vi "CRC16MODBUS.vi"(8 "error in (no error)":errorcluster caption="错误输入（无错误）", 11 "In_Data":u8[](array[numeric]) format="%.0x") -> (0 "error out":errorcluster caption="错误输出", 3 "CRC16":u16 format="%.0x")   [LabVIEW 2015]
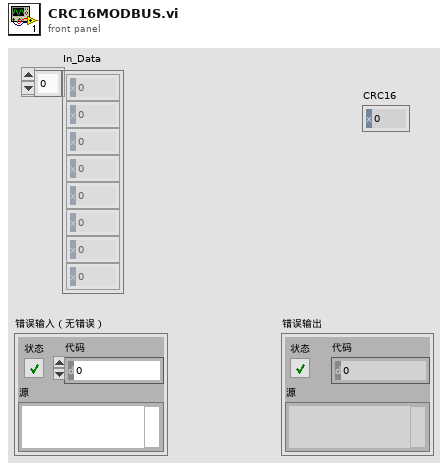
[diagram p1: front panel]
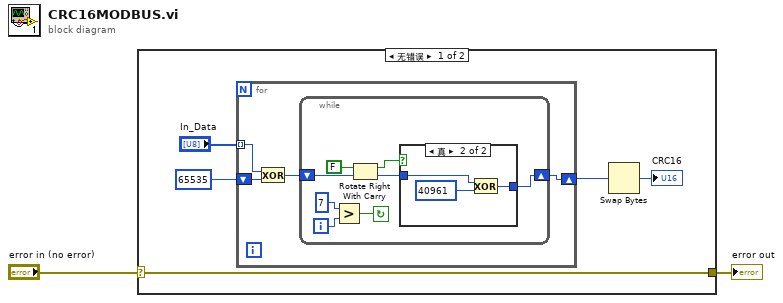
[diagram p0: block diagram]
diagram:
  n1 = case shown="无错误" "error in (no error)" {
    selector: "error in (no error)" -> [w3 w24]
    tunnel: [w3 w24] -> w1
    frame No Error {
      n2 = for {
        tunnel: "In_Data" -> [w11] mode=indexing
        shift-right: [w8] -> w5
        shift-left: 65535 -> [w10]
        n3 = Exclusive Or(1:w10, 2:w11) -> (0:w9:i32)
        n4 = while {
          shift-right: [w15] -> w8
          shift-left: w9 -> [w18]
          i -> [w14]
          stop <- w12 continue-if-true
          n5 = Greater?(x=7, y=w14) -> (0:w12:bool)
          n6 = Rotate Right With Carry(2:w18, 3:FALSE) -> (0:w17:i32, 1:w16:bool)
          n7 = case shown="真" w16 {
            tunnel: w17 -> [w20 w23]
            tunnel: [w20 w21] -> w15
            frame False {
            }
            frame True {
              n8 = Exclusive Or(1:40961, 2:w23) -> (0:w21:i32)
            }
          }
        }
      }
      n9 = Swap Bytes(anything=w5) -> (byte swapped=→"CRC16":i32)
    }
    frame Error {
    }
  }
  "error out" <- w1
